vi "DependencyViewer_Tester.vi"() -> ()   [LabVIEW 2020]
uses:
  DependencyViewer/DependencyViewer/DependencyConfiguration.ctl
  DependencyViewer/DependencyViewer/FilterOptions.ctl
  DependencyViewer/VISJS-Viewer/VISJS Viewer.lvlib
  DependencyViewer/DependencyViewer/DependencyViewer.lvlib
panel:
  in  "Configuration":T1={"Name"="All Project Items", "RemoveItemsBelongingToLibraries"=FALSE, "RemoveEvenSubLibraries"=FALSE, "FilterOptions"={"Ignore user.lib"=TRUE, "Ignore vi.lib"=TRUE, "Ignore instr.lib"=TRUE, "FolderToIgnore"=[], "Ignore libraries"=FALSE, "Ignore lvcasses"=FALSE, "Ignore xnodes"=TRUE, "Ignore xcontrols"=TRUE, "Ignore Channel Classes"=TRUE}, "OnlyKeepCircularDepedencies"=FALSE, "IgnoreLibrariesInCircularDependencies"=FALSE, "Depth"=0}
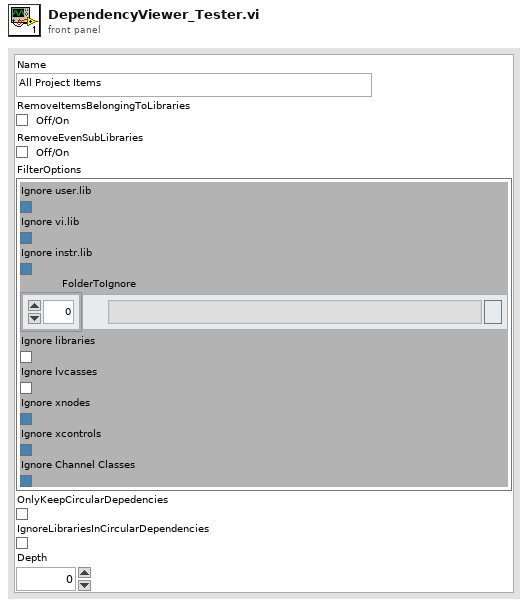
[diagram p1: front panel]
types:
  T1 = typedef "DependencyViewer.lvlib/DependencyConfiguration.ctl" = cluster{"Name":string, "RemoveItemsBelongingToLibraries":bool, "RemoveEvenSubLibraries":bool, "FilterOptions":T2, "OnlyKeepCircularDepedencies":bool, "IgnoreLibrariesInCircularDependencies":bool, "Depth":i32}
  T2 = typedef "DependencyViewer.lvlib/FilterOptions.ctl" = cluster{"Ignore user.lib":bool, "Ignore vi.lib":bool, "Ignore instr.lib":bool, "FolderToIgnore":path[], "Ignore libraries":bool, "Ignore lvcasses":bool, "Ignore xnodes":bool, "Ignore xcontrols":bool, "Ignore Channel Classes":bool}
  T3 = typedef "DependencyViewer.lvlib/LibraryDependentInfo.vi" = cluster{"Type":T4, "Path":path, "FullQualifierName":string, "DependentLibrary":map{path, set{path}}, "ParentLibraries":path[], "IsInterface":bool}
  T4 = typedef "NI_FileType.lvlib/FT_FileTypes.ctl" = enum32{"Invalid file/path", "Unknown type", "Instrument", "Control", "Polymorphic VI", "Project", "Library", "LVClass", "XControl", "XNode", "CIN", "Run-time menu", "Palette menu", "LLB", "Shortcut", "Directory", "Class Private Data Control", "Statechart", "MathScript .m file", "Ladder Diagram", "LVLibp"}
  T5 = typedef "DependencyViewer.lvlib/FileDependencyType.ctl" = cluster{"Path":path, "FileType":T4, "FullQualifierName":string, "OwnerPath":path, "Dependencies":path[], "ParentLibraries":path[], "IsInterface":bool}
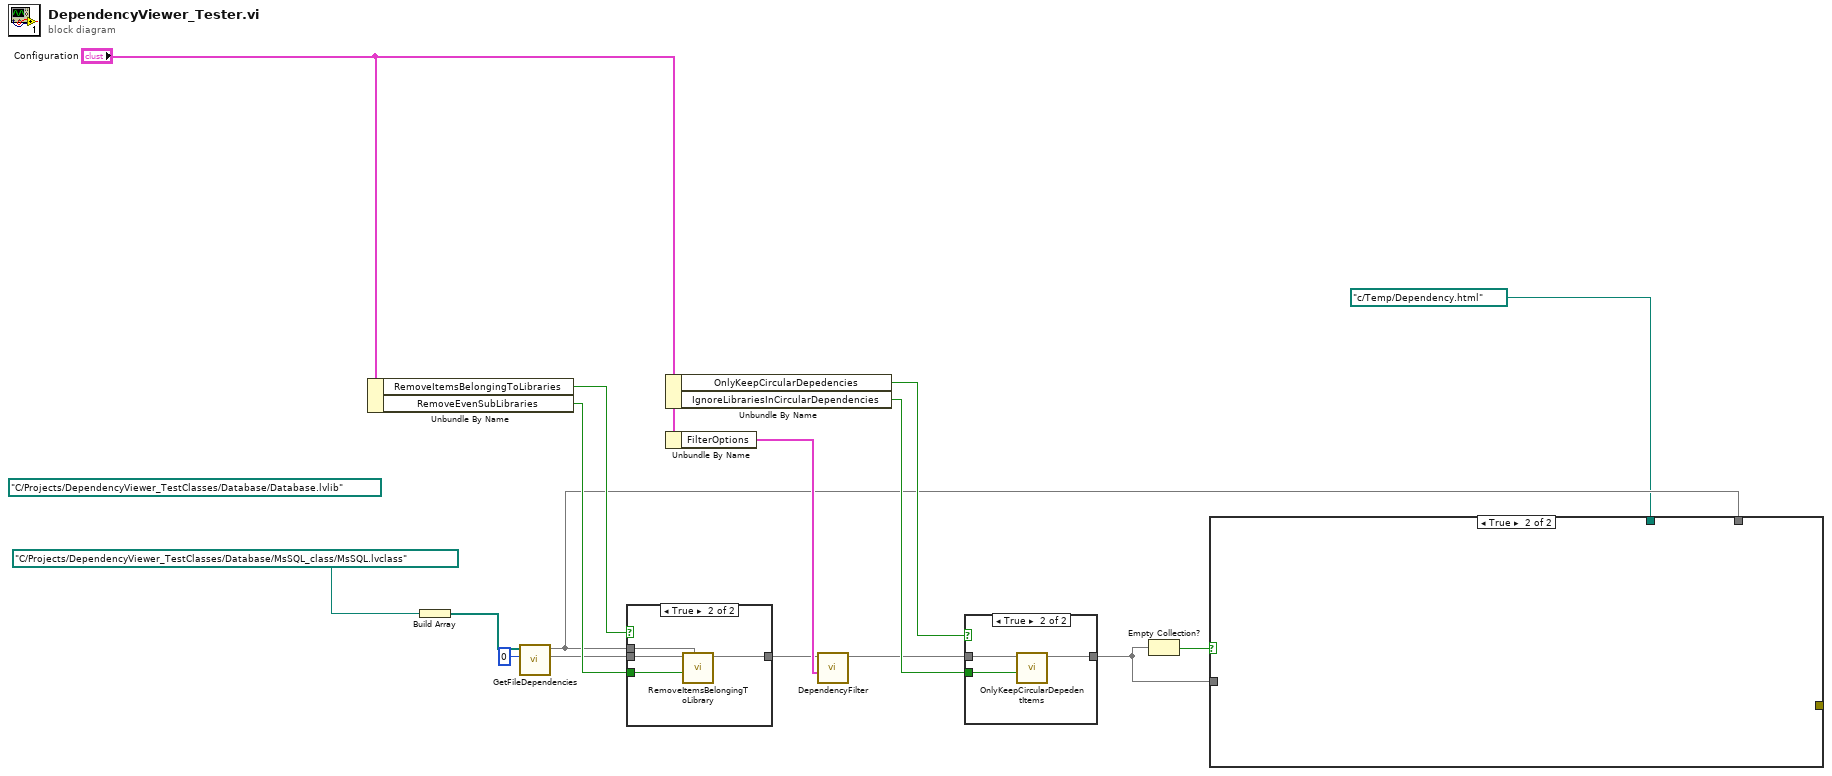
[diagram p0: block diagram]
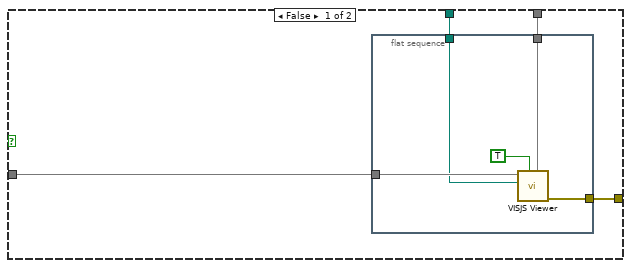
[diagram p4: hidden frame]
diagram:
  (unwired) path "C:/Projects/DependencyViewer_TestClasses/Database/Database.lvlib"
  n1 = Unbundle By Name("Configuration") -> ("RemoveItemsBelongingToLibraries"=w10:bool, "RemoveEvenSubLibraries"=w11:bool)
  n2 = Build Array(path "C:/Projects/DependencyViewer_TestClasses/Database/MsSQL_class/MsSQL.lvclass") -> (w3:path[])
  n3 = call "GetFileDependencies.vi"("MaxDepth(<=0 No limit)"=0, "All Files in Dir"=w3) -> ("LibraryDependency"=w9:map{path, T3}, "FileDependency out"=w6:map{path, T5})  [unwired: 8 in]
  n4 = case shown="True" w10 {
    tunnel: w6 -> [_ w21]
    tunnel: [w17 w20] -> w8
    tunnel: w9 -> [w17 w19]
    tunnel: w11 -> [_ w18]
    frame False {
    }
    frame True {
      n5 = call "RemoveItemsBelongingToLibrary.vi"("FileDependency In"=w21, "EvenSubLibraries"=w18, "LibraryDependency In"=w19) -> ("LibraryDependency Out"=w20:map{path, T3})  [unwired: 8 in]
    }
  }
  n6 = Unbundle By Name("Configuration") -> ("OnlyKeepCircularDepedencies"=w13:bool, "IgnoreLibrariesInCircularDependencies"=w14:bool)
  n7 = Unbundle By Name("Configuration") -> ("FilterOptions"=w12:T2)
  n8 = call "DependencyFilter.vi"("FilterOptions"=w12, "LibraryDependency In"=w8) -> ("Filtered LibraryDependency Out"=w7:map{path, T3})  [unwired: 9 in]
  n9 = case shown="True" w13 {
    tunnel: [w22 w25] -> w15
    tunnel: w7 -> [w22 w24]
    tunnel: w14 -> [_ w23]
    frame False {
    }
    frame True {
      n10 = call "OnlyKeepCircularDepedentItems.vi"("IgnoreLibrariesInCircularDependencies(True)"=w23, "LibraryDependency In"=w24) -> ("LibraryDependency Out"=w25:map{path, T3})  [unwired: 9 in]
    }
  }
  n11 = Empty Collection?(1:w15) -> (0:w16:bool)
  n12 = case shown="True" w16 {
    tunnel: w6 -> [w29 _]
    tunnel: w15 -> [w28 _]
    tunnel: path "c:/Temp/Dependency.html" -> [w27 _]
    tunnel: [w26 _] -> _
    frame False {
      n13 = flat-sequence {
        tunnel: w29 -> [w34]
        tunnel: w28 -> [w32]
        tunnel: w27 -> [w31]
        tunnel: [w30] -> w26
        frame #0 {
          n14 = call "VISJS Viewer.vi"("FileDependency In"=w34, "OpenWebBrowser(False)"=TRUE, "HTMLFilePath"=w31, "LibraryDependency"=w32) -> ("error out"=w30:errorcluster)  [unwired: 6 in, 1 out]
        }
      }
    }
    frame True {
    }
  }
